vi "Meas Result Update Reading Status.vi"(8 "error in":errorcluster, 9 "f [Hz]":dbl, 10 "reading":T1, 11 "str ref":refnum<vi>) -> (0 "error out":errorcluster)   [LabVIEW 2013]
doc: "Updates status line with current reading data."
uses:
  bridge/Bridge Reading Data.ctl
  drivers/TWM client/Meas Proc QWTB Spectrum Data.ctl
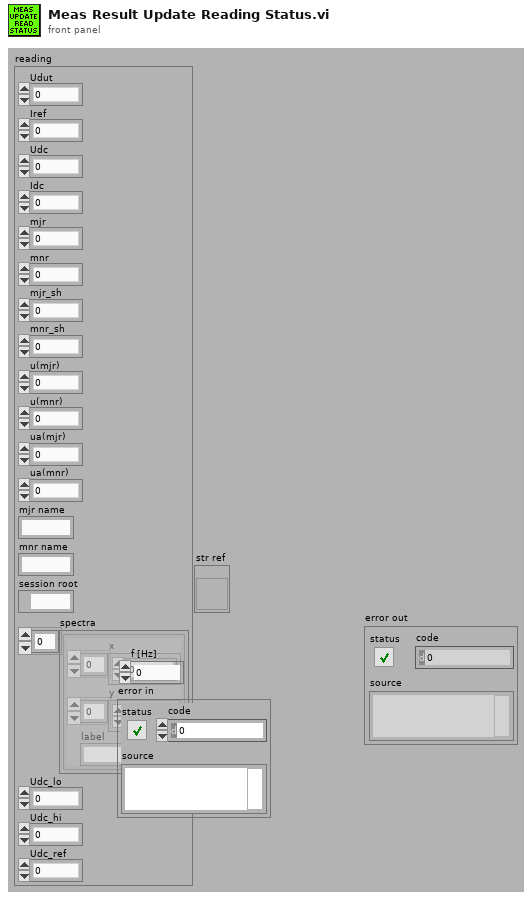
[diagram p1: front panel]
types:
  T1 = typedef "Bridge Reading Data.ctl" = cluster{"Udut":dbl, "Iref":dbl, "Udc":dbl, "Idc":dbl, "mjr":dbl, "mnr":dbl, "mjr_sh":dbl, "mnr_sh":dbl, "u(mjr)":dbl, "u(mnr)":dbl, "ua(mjr)":dbl, "ua(mnr)":dbl, "mjr name":string, "mnr name":string, "session root":path, "spectra":T2[], "Udc_lo":dbl, "Udc_hi":dbl, "Udc_ref":dbl}
  T2 = typedef "Meas Proc QWTB Spectrum Data.ctl" = cluster{"x":sgl[], "y":sgl[], "label":string}
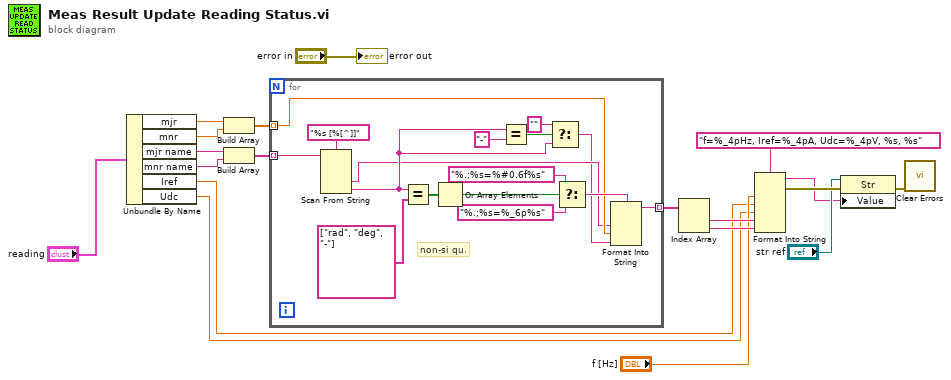
[diagram p0: block diagram]
diagram:
  n1 = Unbundle By Name("reading") -> ("mjr"=w17:dbl, "mnr"=w16:dbl, "mjr name"=w15:string, "mnr name"=w14:string, "Iref"=w7:dbl, "Udc"=w6:dbl)
  n2 = Build Array(w17, w16) -> (w13:dbl[])
  n3 = Build Array(w15, w14) -> (w12:string[])
  n4 = for {
    tunnel: w13 -> [w25] mode=indexing
    tunnel: w12 -> [w35] mode=indexing
    tunnel: [w22] -> w11 mode=indexing
    # "non-si qu."
    n5 = Scan From String(format string="%s [%[^]]", input string=w35) -> (output 1=w24:string, output 2=w28:string)  [unwired: 4 in, 3 out]
    n6 = Equal?(x=w28, y=string[] ["rad", "deg", "-"]) -> (x = y?=w32:bool[])
    n7 = Or Array Elements(Boolean array=w32) -> (logical OR=w31:bool)
    n8 = Equal?(x=w28, y="-") -> (x = y?=w29:bool)
    n9 = Select(t="", s=w29, f=w28) -> (s? t:f=w23:string)
    n10 = Select(t="%.;%s=%#0.6f%s" ("format string"), s=w31, f="%.;%s=%_6p%s" ("format string")) -> (s? t:f=w26:string)
    n11 = Format Into String(format string=w26, w24, w25, w23) -> (resulting string=w22:string)  [unwired: 2 in, 1 out]
  }
  n12 = Index Array(array=w11) -> (element #1=w10:string, element #2=w9:string)  [unwired: 2 in]
  n13 = Format Into String(format string="f=%_4pHz, Iref=%_4pA, Udc=%_4pV, %s, %s", "f [Hz]", w7, w6, w10, w9) -> (resulting string=w2:string, error out=w4:errorcluster)  [unwired: 2 in]
  n14 = property class="Str"(reference="str ref", error in=w4, "Value"=w2) -> (error out=w1:errorcluster)  [unwired: 1 out]
  n15 = call <vilib>:"Clear Errors.vi"("error in (no error)"=w1) -> ()  [unwired: 6 in, 1 out]
  "error out" <- "error in"
